vi "GetMarkerImage.vi"(4 "File type":T1, 5 "Disabled":bool, 7 "image directory":path, 8 "error in":errorcluster, 11 "Knob in":refnum<class "Knob.lvclass">) -> (0 "error out":errorcluster, 3 "Knob out":refnum<class "Knob.lvclass">)   [LabVIEW 2014, in "Knob.lvclass"]
uses:
  Knob.lvclass
  Control/ImageTypes.ctl
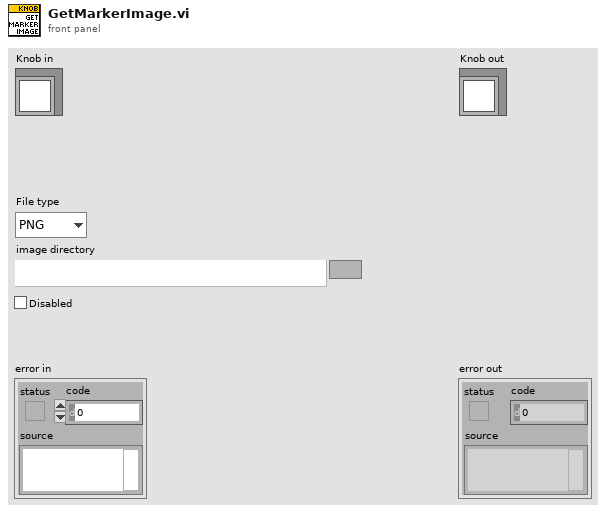
[diagram p1: front panel]
types:
  T1 = typedef "ImageTypes.ctl" = enum16{"PNG", "JPEG", "BMP"}
  T2 = typedef "imagedata.ctl" = cluster{"image type":i32, "image depth":i32, "image":u8[], "mask":u8[], "colors":u32[], "Rectangle":cluster{"left":i16, "top":i16, "right":i16, "bottom":i16}}
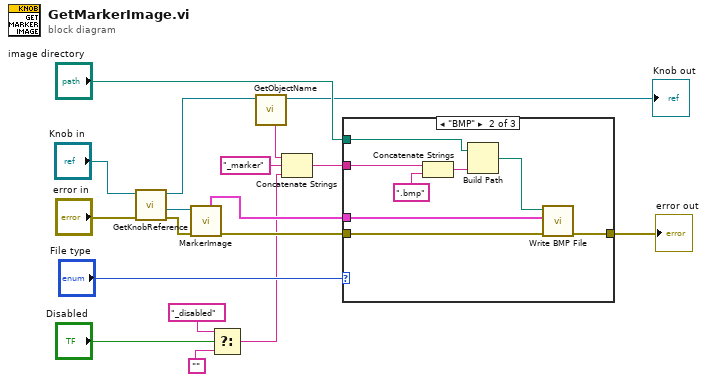
[diagram p0: block diagram]
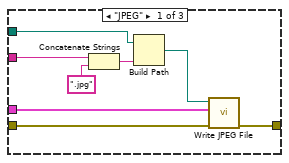
[diagram p2: hidden frame]
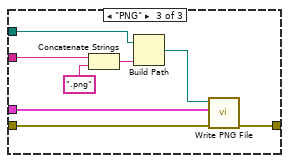
[diagram p3: hidden frame]
diagram:
  n1 = call "GetKnobReference.vi"("error in"="error in", "Knob in"="Knob in") -> ("error out"=w7:errorcluster, "knob reference"=w8:refnum<vi>, "Knob out"=w9:refnum<class "Knob.lvclass">)  [unwired: 7 in]
  n2 = call "MarkerImage.vi"("error in"=w7, "knob"=w8) -> ("error out"=w6:errorcluster, "marker"=w5:T2)  [unwired: 5 in, 1 out]
  n3 = Select(t="_disabled", s="Disabled", f="") -> (s? t:f=w1:string)
  n4 = call-dynamic "GetObjectName.vi"("GObject in"=w9) -> ("GObject out"=→"Knob out":refnum<class "Knob.lvclass">, "Name"=w14:string)  [unwired: 6 in, 1 out]
  n5 = Concatenate Strings(w14, "_marker" ("string"), w1) -> (w12:string)
  n6 = case shown="\"BMP\"" "File type" {
    tunnel: w5 -> [w26 w34 w42]
    tunnel: [w25 w33 w41] -> w11
    tunnel: w6 -> [w24 w32 w40]
    tunnel: w12 -> [w23 w31 w39]
    tunnel: "image directory" -> [w19 w27 w35]
    frame "JPEG" {
      n7 = Concatenate Strings(w23, ".jpg" ("string")) -> (w21:string)
      n8 = Build Path(base path=w19, name or relative path=w21) -> (appended path=w20:path)
      n9 = call <vilib>:"Write JPEG File.vi"("error in (no error)"=w24, "image data"=w26, "path to JPEG file"=w20) -> ("error out"=w25:errorcluster)  [unwired: 7 in, 1 out]
    }
    frame "BMP" {
      n10 = Concatenate Strings(w31, ".bmp" ("string")) -> (w29:string)
      n11 = Build Path(base path=w27, name or relative path=w29) -> (appended path=w28:path)
      n12 = call <vilib>:"Write BMP File.vi"("error in (no error)"=w32, "image data"=w34, "path to BMP file"=w28) -> ("error out"=w33:errorcluster)  [unwired: 7 in, 1 out]
    }
    frame "PNG" {
      n13 = Concatenate Strings(w39, ".png" ("string")) -> (w37:string)
      n14 = Build Path(base path=w35, name or relative path=w37) -> (appended path=w36:path)
      n15 = call <vilib>:"Write PNG File.vi"("error in (no error)"=w40, "image data"=w42, "path to PNG file"=w36) -> ("error out"=w41:errorcluster)  [unwired: 7 in, 1 out]
    }
  }
  "error out" <- w11
